vi "Alarms Display.vi"(4 "Alarm Input":bool, 6 "Fault Input":bool, 8 "Error In":errorcluster, 11 "Alarms Data In":T2) -> (0 "Error Out":errorcluster, 1 "Alarm?":bool, 2 "Fault?":bool, 3 "Alarm List":T1)   [LabVIEW 2014]
uses:
  Controls/Alarms Data.ctl
  Controls/Alarm Display.ctl
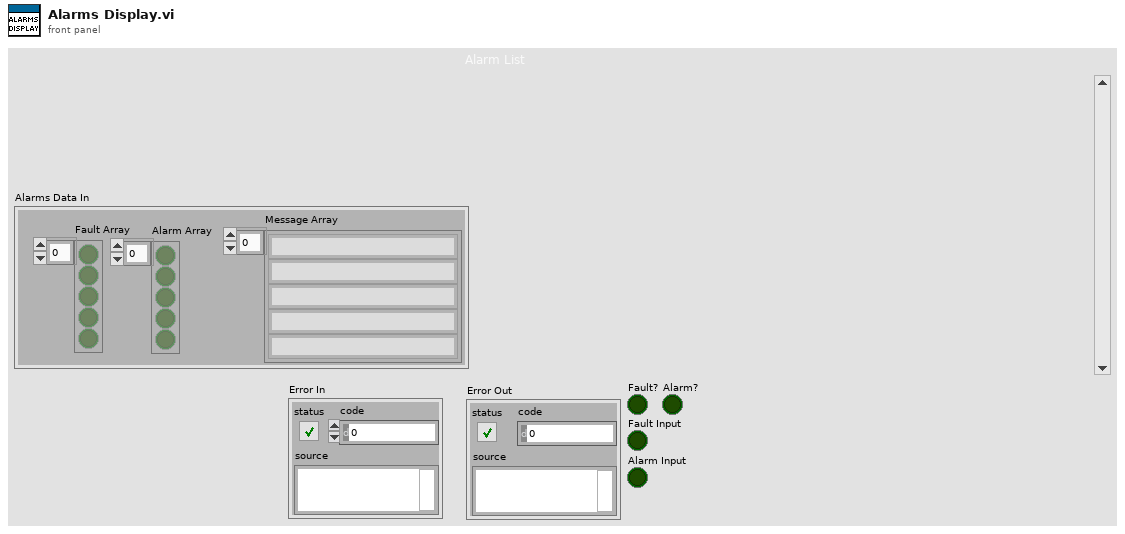
[diagram p1: front panel]
types:
  T1 = typedef "Alarm Display.ctl" = string[]
  T2 = typedef "Alarms Data.ctl" = cluster{"Message Array":string[], "Fault Array":bool[], "Alarm Array":bool[]}
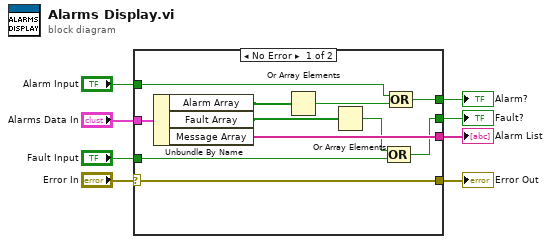
[diagram p0: block diagram]
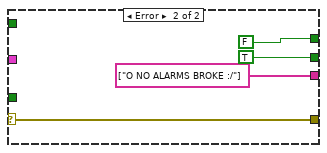
[diagram p2: hidden frame]
diagram:
  n1 = case shown="No Error" "Error In" {
    selector: "Error In" -> [w19 w23]
    tunnel: [w19 w23] -> w7
    tunnel: "Alarms Data In" -> [w18 _]
    tunnel: [w17 string[] ["O NO ALARMS BROKE :/"] ("Message Array")] -> w5
    tunnel: [w13 TRUE] -> w4
    tunnel: [w11 FALSE] -> w3
    tunnel: "Fault Input" -> [w12 _]
    tunnel: "Alarm Input" -> [w9 _]
    frame No Error {
      n2 = Unbundle By Name(w18) -> ("Alarm Array"=w16:bool[], "Fault Array"=w15:bool[], "Message Array"=w17:string[])
      n3 = Or Array Elements(Boolean array=w16) -> (logical OR=w10:bool)
      n4 = Or Array Elements(Boolean array=w15) -> (logical OR=w14:bool)
      n5 = Compound Arithmetic op=OR(w14, w12) -> (w13:bool)
      n6 = Compound Arithmetic op=OR(w9, w10) -> (w11:bool)
    }
    frame Error {
    }
  }
  "Error Out" <- w7
  "Alarm List" <- w5
  "Fault?" <- w4
  "Alarm?" <- w3
